vi "用户登录数据库解析.vi"(11 "text":string) -> (1 "异常信息":string, 3 "权限":string)   [LabVIEW 2014]
panel:
  out "roles":string[](array[string])
  out "code":i32
  out "msg":string
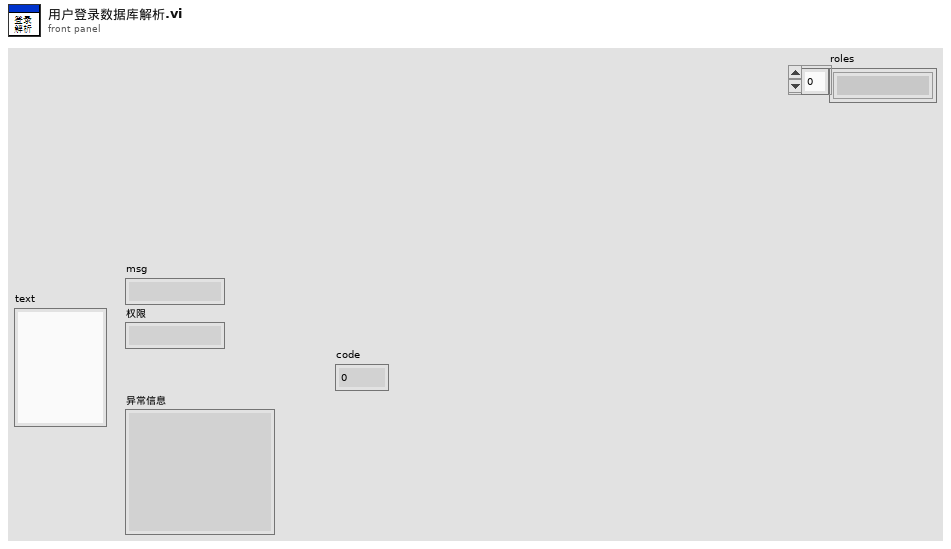
[diagram p1: front panel]
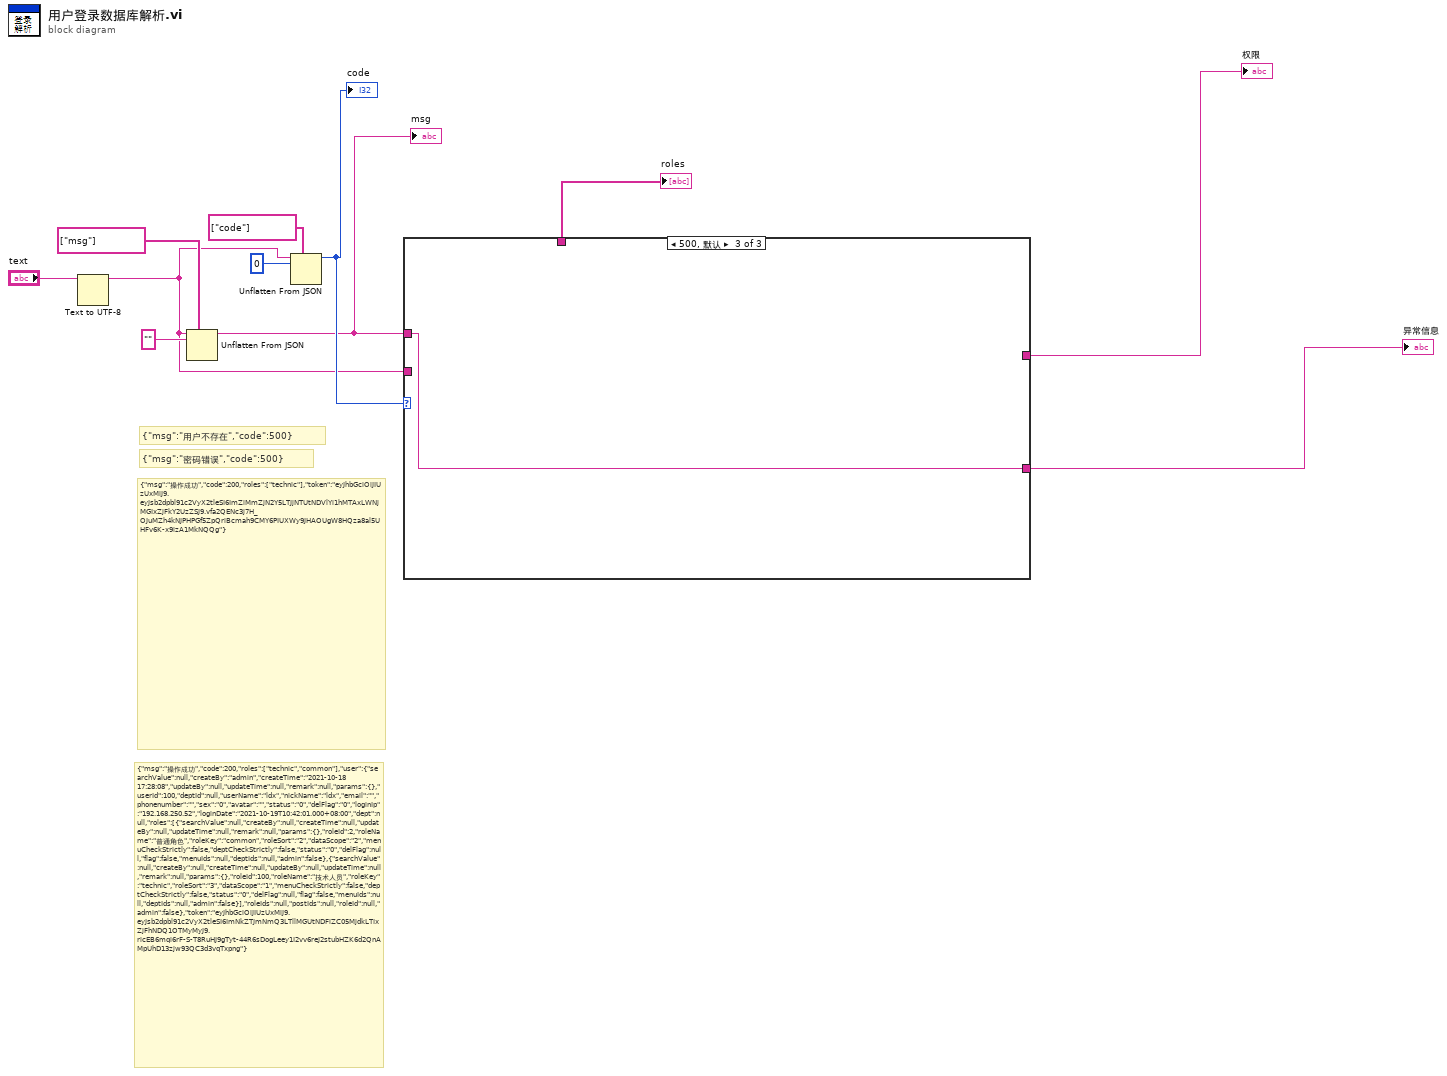
[diagram p0: block diagram]
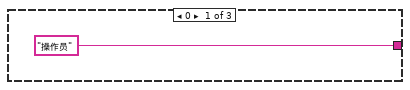
[diagram p2: hidden frame]
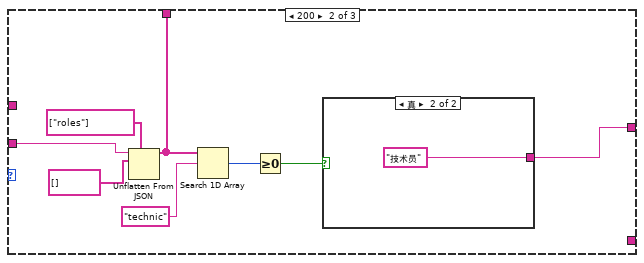
[diagram p3: hidden frame]
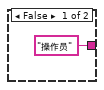
[diagram p4: hidden frame]
diagram:
  # "{\"msg\":\"操作成功\",\"code\":200,\"roles\":[\"technic\",\"common\"],\"user\":{\"searchValue\":null,\"createBy\":\"admin\",\"createTime\":\"2021-10-18 17:28:08\",\"updateBy\":null,\"updateTime\":null,\"remark\":null,\"params\":{},\"userId\":100,\"deptId\":null,\"userName\":\"ldx\",\"nickName\":\"ldx\",\"email\":\"\",\"phonenumber\":\"\",\"sex\":\"0\",\"avatar\":\"\",\"status\":\"0\",\"delFlag\":\"0\",\"loginIp\":\"192.168.250.52\",\"loginDate\":\"2021-10-19T10:42:01.000+08:00\",\"dept\":null,\"roles\":[{\"searchValue\":null,\"createBy\":null,\"createTime\":null,\"updateBy\":null,\"updateTime\":null,\"remark\":null,\"params\":{},\"roleId\":2,\"roleName\":\"普通角色\",\"roleKey\":\"common\",\"roleSort\":\"2\",\"dataScope\":\"2\",\"menuCheckStrictly\":false,\"deptCheckStrictly\":false,\"status\":\"0\",\"delFlag\":null,\"flag\":false,\"menuIds\":null,\"deptIds\":null,\"admin\":false},{\"searchValue\":null,\"createBy\":null,\"createTime\":null,\"updateBy\":null,\"updateTime\":null,\"remark\":null,\"params\":{},\"roleId\":100,\"roleName\":\"技术人员\",\"roleKey\":\"technic\",\"roleSort\":\"3\",\"dataScope\":\"1\",\"menuCheckStrictly\":false,\"deptCheckStrictly\":false,\"status\":\"0\",\"delFlag\":null,\"flag\":false,\"menuIds\":null,\"deptIds\":null,\"admin\":false}],\"roleIds\":null,\"postIds\":null,\"roleId\":null,\"admin\":false},\"token\":\"eyJhbGciOiJIUzUxMiJ9.eyJsb2dpbl91c2VyX2tleSI6ImNkZTJmNmQ3LTllMGUtNDFiZC05MjdkLTIxZjFhNDQ1OTMyMyJ9.ricEB6mqi6rF-S-T8RuHJ9gTyt-44R6sDogLeey1I2vv6reJ2stubHZK6d2QnAMpUhD13zjw93QC3d3vqTxpng\"}"
  # "{\"msg\":\"操作成功\",\"code\":200,\"roles\":[\"technic\"],\"token\":\"eyJhbGciOiJIUzUxMiJ9.eyJsb2dpbl91c2VyX2tleSI6ImZiMmZjN2Y5LTJjNTUtNDVlYi1hMTAxLWNjMGIxZjFkY2UzZSJ9.vfa2QENc3j7H_OJuMZh4kNJPHPGf5ZpQriBcmah9CMY6PIUXWy9JHAOUgW8HQza8al5UHFv6K-x9izA1MkNQQg\"}"
  # "{\"msg\":\"密码错误\",\"code\":500}"
  # "{\"msg\":\"用户不存在\",\"code\":500}"
  n1 = Text to UTF-8(11:"text") -> (3:w3:string)  [unwired: 2 in, 1 out]
  n2 = Unflatten From JSON(path=string[] ["msg"], JSON string=w3, type and defaults="") -> (value=w2:string)  [unwired: 4 in, 1 out]
  "msg" <- w2
  n3 = Unflatten From JSON(path=string[] ["code"], JSON string=w3, type and defaults=0) -> (value=w4:i32)  [unwired: 4 in, 1 out]
  "code" <- w4
  n4 = case shown="500, 默认" w4 {
    tunnel: ["操作员" w20 _] -> w11
    tunnel: [_ _ w23] -> w10
    tunnel: w3 -> [_ w18 _]
    tunnel: w2 -> [_ _ w23]
    tunnel: [_ w13 _] -> w1
    frame 0 {
    }
    frame 200 {
      n5 = Unflatten From JSON(path=string[] ["roles"], JSON string=w18, type and defaults=string[] []) -> (value=w13:string[])  [unwired: 4 in, 1 out]
      n6 = Search 1D Array(1D array=w13, element="technic" ("搜索字符串")) -> (index of element=w15:i32)  [unwired: 1 in]
      n7 = Greater Or Equal To 0?(x=w15) -> (x >= 0?=w14:bool)
      n8 = case shown="真" w14 {
        tunnel: ["操作员" "技术员"] -> w20
        frame False {
        }
        frame True {
        }
      }
    }
    frame 500, Default {
    }
  }
  "权限" <- w11
  "异常信息" <- w10
  "roles" <- w1
